vi "16-ParseSubPacketsByNumber.vi"(10 "Number of Sub Packets":u32, 11 "BITS in":bool[](array[boolean])) -> (2 "Sub Packets":T1(array[cluster]), 3 "BITS out":bool[](array[boolean]))   [LabVIEW 2019, in "16.lvlib"]
uses:
  16.lvlib
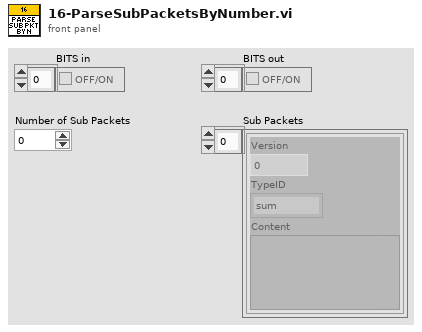
[diagram p1: front panel]
types:
  T1 = cluster{"Version":u32, "TypeID":enum16{"sum", "product", "minimum", "maximum", "literal", "greater than", "less than", "equal to"}, "Content":variant}[]
  T2 = cluster{"Version":u32, "TypeID":enum16{"sum", "product", "minimum", "maximum", "literal", "greater than", "less than", "equal to"}, "Content":variant}
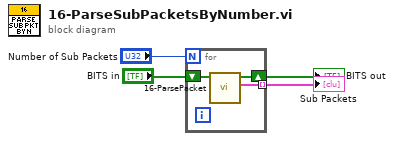
[diagram p0: block diagram]
diagram:
  n1 = for {
    N: "Number of Sub Packets" -> [_]
    tunnel: [w7] -> w4 mode=indexing
    shift-right: [w5] -> w3
    shift-left: "BITS in" -> [w6]
    n2 = call "16-ParsePacket.vi"("BITS in"=w6) -> ("Packet"=w7:T2, "BITS out"=w5:bool[])  [unwired: 9 in]
  }
  "Sub Packets" <- w4
  "BITS out" <- w3
